vi "获取量程参数存入关键参数.vi"(7 "关键参数变更":bool, 8 "error in (no error)":errorcluster caption="错误输入（无错误）", 9 "量程":u16, 10 "flowid":u16, 11 "id":u16) -> (0 "error out":errorcluster caption="错误输出")   [LabVIEW 2016, in "斯坦道总磷总氮.lvlib"]
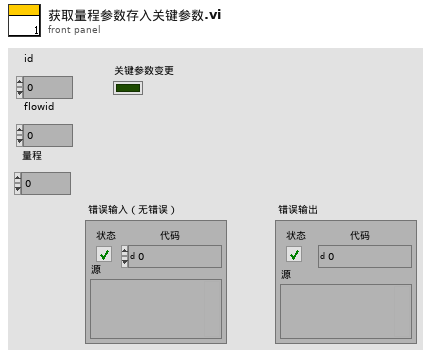
[diagram p1: front panel]
types:
  T1 = cluster{"运行模式":enum16{"维护模式", "常规模式", "应急模式", "质控模式", "性能测试"}, "质控频次":enum16{"关闭", "每天", "星期一", "星期二", "星期三", "星期四", "星期五", "星期六", "星期日"}, "空白核查时间":u16, "跨度核查时间":u16, "测量间隔":u16}
  T2 = cluster{"总磷":dbl, "总氮":dbl, "氨氮":dbl, "磷酸盐":dbl, "硝氮":dbl, "亚硝氮":dbl, "硅酸盐":dbl, "硫化物":dbl, "COD":dbl, "氟化物":dbl, "CODMn":dbl}
  T3 = cluster{"标液浓度1":dbl, "测量吸光度1":dbl, "样品1启用":bool, "标液浓度2":dbl, "测量吸光度2":dbl, "样品2启用":bool, "标液浓度3":dbl, "测量吸光度3":dbl, "样品3启用":bool, "标液浓度4":dbl, "测量吸光度4":dbl, "样品4启用":bool, "标液浓度5":dbl, "测量吸光度5":dbl, "样品5启用":bool, "模型":enum32{"线性", "多项式"}, "精度":dbl, "XY图":cluster{"X Values":dbl[], "Y Values":dbl[]}[], "拟合公式":string, "r^2":dbl, "标样一校准时间":timestamp, "标样二校准时间":timestamp, "标样三校准时间":timestamp, "标样四校准时间":timestamp, "标样五校准时间":timestamp, "二次方程":cluster{"c":dbl, "x":dbl, "x^2":dbl}, "标定时间":timestamp}
  T4 = cluster{"测量精度":u16, "检出限":dbl, "上限":dbl, "下限":dbl, "阈值（低->高）":dbl, "阈值（高->低）":dbl, "稀释度":dbl}
  T5 = typedef "SingleStepTestV3.lvlib/SingleStepTestV3.lvclass/仪器版本.ctl" = enum16{"V3.1版", "V4版", "V3版", "V4.2版"}
  T6 = typedef "斯坦道总磷总氮.lvlib/V3.1版外设参数.ctl" = cluster{"泵类型":u8, "进样速度":u32, "出样速度":u32, "泵阀量":u8, "阀方向":u8, "光谱仪类型":u8, "光谱采样次数":u8, "氙灯次数":u8, "B":u16, "C":u16, "D":u16, "E":u16, "B_COD":u16, "C_COD":u16, "D_COD":u16, "E_COD":u16, "G":u16, "M":u16, "N":u16, "氨氮注射泵控温下限":sgl, "氨氮注射泵控温上限":sgl, "总氮注射泵控温下限":sgl, "总氮注射泵控温上限":sgl, "消解温度下限":sgl, "消解温度上限":sgl, "加热10s限值":sgl, "KP":sgl, "KI":sgl, "KD":sgl, "高温高压阀开阀温度":sgl, "总氮x公式0":u8, "总氮x公式1":sgl, "总氮x公式2":sgl, "总磷浊度稀释系数":sgl, "总磷浊度补偿权重1":sgl, "总磷浊度补偿权重2":sgl, "盐度系数":sgl, "氨氮补偿系数1":sgl, "氨氮补偿系数2":sgl}
  T7 = typedef "斯坦道总磷总氮.lvlib/V4版外设参数.ctl" = cluster{"泵类型":u8, "注射泵正常速度":u32, "注射泵慢速":u32, "阀型号":u8, "res":u8, "光谱仪类型":u8, "光谱采样次数":u8, "氙灯次数":u8, "B":u16, "C":u16, "D":u16, "E":u16, "B_COD":u16, "C_COD":u16, "D_COD":u16, "E_COD":u16, "G":u16, "M":u16, "N":u16, "降温下限":sgl, "降温上限":sgl, "恒温温度下限":sgl, "恒温温度上限":sgl, "消解温度下限":sgl, "消解温度上限":sgl, "加热10s限值":sgl, "KP":sgl, "KI":sgl, "KD":sgl, "高温高压阀开阀温度":sgl, "总氮x公式0":u8, "总氮x公式1":sgl, "总氮x公式2":sgl, "总磷浊度稀释系数":sgl, "总磷浊度补偿权重1":sgl, "总磷浊度补偿权重2":sgl, "盐度系数":sgl, "氨氮补偿系数1":sgl, "氨氮补偿系数2":sgl, "缺试剂传感器阈值":u16}
  T8 = typedef "斯坦道总磷总氮.lvlib/V4.2版外设参数.ctl" = cluster{"工作模式":u16, "泵类型":u16, "阀型号":u16, "注射泵进样速度":u16, "注射泵出样速度":u16, "注射泵滴定速度":u16, "res":u16, "注射泵慢速":u16, "光谱仪类型":u16, "光谱采样次数":u16, "氙灯次数":u16, "B":u16, "C":u16, "D":u16, "E":u16, "B_COD":u16, "C_COD":u16, "D_COD":u16, "E_COD":u16, "G":u16, "M":u16, "N":u16, "温度校准参数":sgl, "降温温度":sgl, "恒温温度":sgl, "消解温度":sgl, "高温高压阀开阀温度":sgl, "加热超时时间":sgl, "KP":sgl, "KI":sgl, "KD":sgl, "消解PID积分上限":sgl, "恒温PID积分上限":sgl, "PID积分下限":sgl, "缺试剂传感器阈值":u16, "滴定延时":u16, "滴定斜率阈值":sgl, "总氮x公式0":u16, "总氮x公式1":sgl, "总氮x公式2":sgl, "总磷浊度稀释系数":sgl, "总磷浊度补偿权重1":sgl, "总磷浊度补偿权重2":sgl, "盐度系数":sgl, "氨氮补偿系数1":sgl, "氨氮补偿系数2":sgl}
  T9 = typedef "斯坦道总磷总氮.lvlib/V3版外设参数.ctl" = cluster{"泵类型":u8, "进样速度":u32, "出样速度":u32, "泵阀量":u8, "光谱仪类型":u8, "光谱采样次数":u8, "氙灯次数":u8, "B":u16, "C":u16, "D":u16, "E":u16, "B_COD":u16, "C_COD":u16, "D_COD":u16, "E_COD":u16, "G":u16, "M":u16, "N":u16, "氨氮注射泵控温下限":sgl, "氨氮注射泵控温上限":sgl, "总氮注射泵控温下限":sgl, "总氮注射泵控温上限":sgl, "消解温度下限":sgl, "消解温度上限":sgl, "加热10s限值":sgl, "高温高压阀开阀温度":sgl, "总氮x公式0":u8, "总氮x公式1":sgl, "总氮x公式2":sgl, "总磷浊度稀释系数":sgl, "总磷浊度补偿权重1":sgl, "总磷浊度补偿权重2":sgl, "盐度系数":sgl, "氨氮补偿系数1":sgl, "氨氮补偿系数2":sgl}
  T10 = cluster{"标液浓度1":dbl, "测量吸光度1":dbl, "样品1启用":bool, "标液浓度2":dbl, "测量吸光度2":dbl, "样品2启用":bool, "标液浓度3":dbl, "测量吸光度3":dbl, "样品3启用":bool, "标液浓度4":dbl, "测量吸光度4":dbl, "样品4启用":bool, "标液浓度5":dbl, "测量吸光度5":dbl, "样品5启用":bool, "模型":enum32{"线性", "多项式"}, "精度":dbl, "XY图":cluster{"X Values":dbl[], "Y Values":dbl[]}[], "拟合公式":string, "r^2":dbl, "标样一校准时间":timestamp, "标样二校准时间":timestamp, "标样三校准时间":timestamp, "标样四校准时间":timestamp, "标样五校准时间":timestamp, "二次方程":cluster{"c":dbl, "x":dbl, "x^2":dbl}, "标定时间":timestamp}[]
  T11 = typedef "斯坦道总磷总氮.lvlib/关键参数.ctl" = cluster{"测量量程":sgl, "测量检出限":sgl, "测量精度":sgl, "测量间隔":sgl, "消解温度":sgl, "消解时长":sgl, "三项式系数":sgl, "二次多项式系数":sgl, "曲线斜率":sgl, "曲线截距":sgl, "线性相关系数":sgl, "空白校准时间":timestamp, "标样校准时间":timestamp, "测量信号值":sgl, "稀释倍数":sgl, "空白标定系数":sgl, "量程系数":sgl}
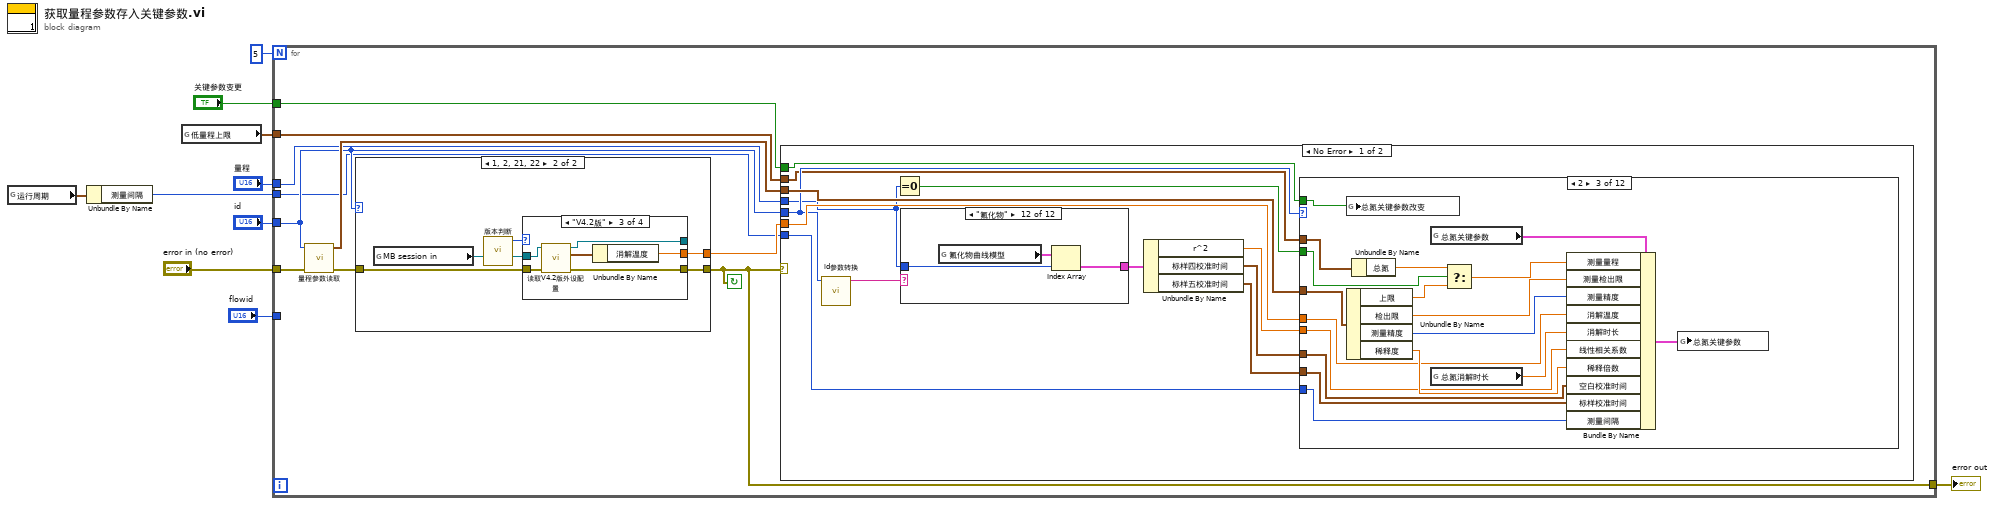
[diagram p0: block diagram]
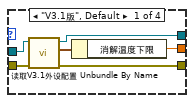
[diagram p3: hidden frame]
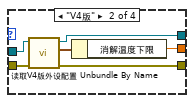
[diagram p4: hidden frame]
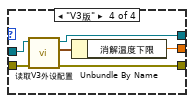
[diagram p5: hidden frame]
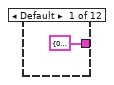
[diagram p6: hidden frame]
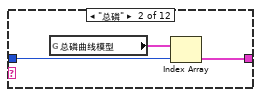
[diagram p7: hidden frame]
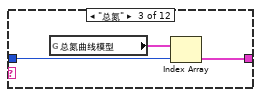
[diagram p8: hidden frame]
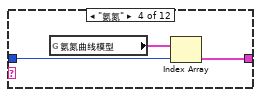
[diagram p9: hidden frame]
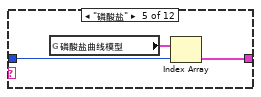
[diagram p10: hidden frame]
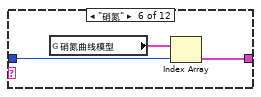
[diagram p11: hidden frame]
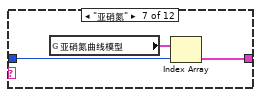
[diagram p12: hidden frame]
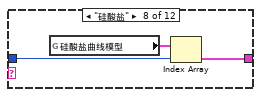
[diagram p13: hidden frame]
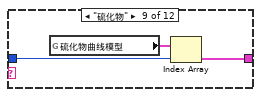
[diagram p14: hidden frame]
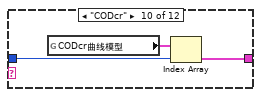
[diagram p15: hidden frame]
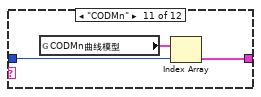
[diagram p16: hidden frame]
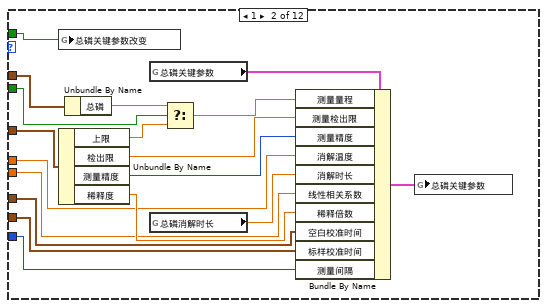
[diagram p18: hidden frame]
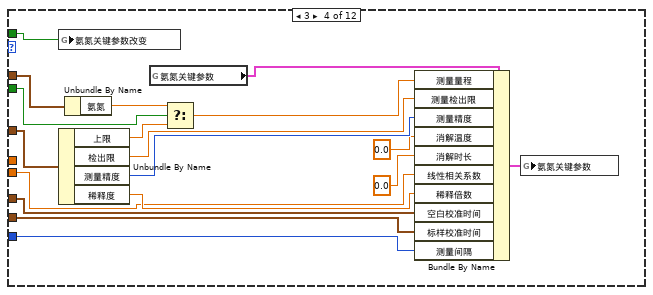
[diagram p19: hidden frame]
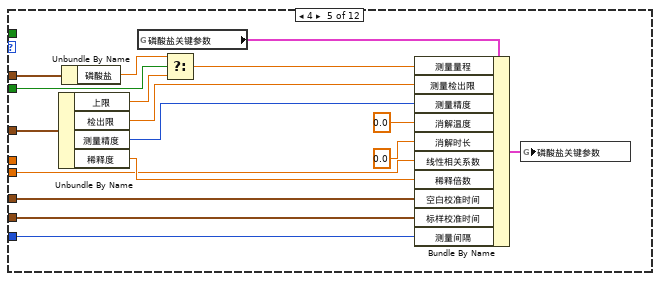
[diagram p20: hidden frame]
diagram:
  n1 = global read "总磷总氮断电保存全局变量.vi" "运行周期"() -> (w4:T1)
  n2 = Unbundle By Name(w4) -> ("测量间隔"=w3:u16)
  n3 = global read "总磷总氮断电保存全局变量.vi" "低量程上限"() -> (w2:T2)
  n4 = for {
    N: 5 -> [_]
    tunnel: "量程" -> [w18]
    tunnel: "flowid" -> [_]
    tunnel: "id" -> [w14]
    tunnel: "error in (no error)" -> [w15]
    tunnel: [w16] -> w5
    tunnel: w3 -> [w13]
    tunnel: w2 -> [w12]
    tunnel: "关键参数变更" -> [w11]
    stop <- w16 continue-if-true
    n5 = call "量程参数读取.vi"("error in (no error)"=w15, "测量参数"=w14) -> ("error out"=w17:errorcluster, "量程参数读取"=w20:T4)  [unwired: 8 in]
    n6 = case shown="1, 2, 21, 22" w14 {
      tunnel: [_ w24] -> w19
      tunnel: w17 -> [w21 w25]
      tunnel: [w21 w23] -> w16
      frame 0, Default {
      }
      frame 1, 2, 21, 22 {
        n7 = global read "VAR总磷总氮全局变量.vi" "MB session in"() -> (w26:refnum<class "MB_Master.lvclass">)
        n8 = call "版本判断.vi"() -> ("仪器版本"=w22:T5)  [unwired: 11 in]
        n9 = case shown="\"V4.2版\"" w22 {
          tunnel: [w32 w38 w44 w50] -> w23
          tunnel: [w30 w36 w42 w48] -> w24
          tunnel: [w29 w35 w41 w47] -> _
          tunnel: w26 -> [w28 w34 w40 w46]
          tunnel: w25 -> [w27 w33 w39 w45]
          frame "V3.1版", Default {
            n10 = call "读取V3.1外设配置.vi"("error in (no error)"=w27, "MB session in"=w28) -> ("error out"=w32:errorcluster, "外设配置"=w31:T6, "MB session out"=w29:refnum<class "MB_Master.lvclass">)  [unwired: 7 in]
            n11 = Unbundle By Name(w31) -> ("消解温度下限"=w30:sgl)
          }
          frame "V4版" {
            n12 = call "读取V4版外设配置.vi"("error in (no error)"=w33, "MB session in"=w34) -> ("error out"=w38:errorcluster, "外设配置"=w37:T7, "MB session out"=w35:refnum<class "MB_Master.lvclass">)  [unwired: 7 in]
            n13 = Unbundle By Name(w37) -> ("消解温度下限"=w36:sgl)
          }
          frame "V4.2版" {
            n14 = call "读取V4.2版外设配置.vi"("error in (no error)"=w39, "MB session in"=w40) -> ("error out"=w44:errorcluster, "外设配置"=w43:T8, "MB session out"=w41:refnum<class "MB_Master.lvclass">)  [unwired: 7 in]
            n15 = Unbundle By Name(w43) -> ("消解温度"=w42:sgl)
          }
          frame "V3版" {
            n16 = call "读取V3外设配置.vi"("error in (no error)"=w45, "MB session in"=w46) -> ("error out"=w50:errorcluster, "外设配置"=w49:T9, "MB session out"=w47:refnum<class "MB_Master.lvclass">)  [unwired: 7 in]
            n17 = Unbundle By Name(w49) -> ("消解温度下限"=w48:sgl)
          }
        }
      }
    }
    n18 = case shown="No Error" w16 {
      tunnel: w20 -> [w63 _]
      tunnel: w19 -> [w62 _]
      tunnel: w14 -> [w56 _]
      tunnel: w18 -> [w53 _]
      tunnel: w13 -> [w55 _]
      tunnel: w12 -> [w54 _]
      tunnel: w11 -> [w51 _]
      frame No Error {
        n19 = call "id参数转换.vi"("id"=w56) -> ("table输出"=w61:string)  [unwired: 9 in, 1 out]
        n20 = Equal To 0?(x=w53) -> (x = 0?=w52:bool)
        n21 = case shown="\"氟化物\"" w61 {
          tunnel: w53 -> [_ w65 w68 w71 w74 w77 w80 w83 w86 w89 w92 w95]
          tunnel: [T3 {"标液浓度1"=0.0, "测量吸光度1"=0.0, "样品1启用"=FALSE, "标液浓度2"=0.0, "测量吸光度2"=0.0, "样品2启用"=FALSE, "标液浓度3"=0.0, "测量吸光度3"=0.0, "样品3启用"=FALSE, "标液浓度4"=0.0, "测量吸光度4"=0.0, "样品4启用"=FALSE, "标液浓度5"=0.0, "测量吸光度5"=0.0, "样品5启用"=FALSE, "模型"=enum."线性", "精度"=0.0, "XY图"=[], "拟合公式"="", "r^2"=0.0, "标样一校准时间"=timestamp(0 s since 1904-01-01), "标样二校准时间"=timestamp(0 s since 1904-01-01), "标样三校准时间"=timestamp(0 s since 1904-01-01), "标样四校准时间"=timestamp(0 s since 1904-01-01), "标样五校准时间"=timestamp(0 s since 1904-01-01), "二次方程"={"c"=0.0, "x"=0.0, "x^2"=0.0}, "标定时间"=timestamp(0 s since 1904-01-01)} ("总磷曲线模型") w66 w69 w72 w75 w78 w81 w84 w87 w90 w93 w96] -> w60
          frame Default {
          }
          frame "总磷" {
            n22 = global read "校准数据全局变量.vi" "总磷曲线模型"() -> (w67:T10)
            n23 = Index Array(array=w67, index=w65) -> (element=w66:T3)
          }
          frame "总氮" {
            n24 = global read "校准数据全局变量.vi" "总氮曲线模型"() -> (w70:T10)
            n25 = Index Array(array=w70, index=w68) -> (element=w69:T3)
          }
          frame "氨氮" {
            n26 = global read "校准数据全局变量.vi" "氨氮曲线模型"() -> (w73:T10)
            n27 = Index Array(array=w73, index=w71) -> (element=w72:T3)
          }
          frame "磷酸盐" {
            n28 = global read "校准数据全局变量.vi" "磷酸盐曲线模型"() -> (w76:T10)
            n29 = Index Array(array=w76, index=w74) -> (element=w75:T3)
          }
          frame "硝氮" {
            n30 = global read "校准数据全局变量.vi" "硝氮曲线模型"() -> (w79:T10)
            n31 = Index Array(array=w79, index=w77) -> (element=w78:T3)
          }
          frame "亚硝氮" {
            n32 = global read "校准数据全局变量.vi" "亚硝氮曲线模型"() -> (w82:T10)
            n33 = Index Array(array=w82, index=w80) -> (element=w81:T3)
          }
          frame "硅酸盐" {
            n34 = global read "校准数据全局变量.vi" "硅酸盐曲线模型"() -> (w85:T10)
            n35 = Index Array(array=w85, index=w83) -> (element=w84:T3)
          }
          frame "硫化物" {
            n36 = global read "校准数据全局变量.vi" "硫化物曲线模型"() -> (w88:T10)
            n37 = Index Array(array=w88, index=w86) -> (element=w87:T3)
          }
          frame "CODcr" {
            n38 = global read "校准数据全局变量.vi" "CODcr曲线模型"() -> (w91:T10)
            n39 = Index Array(array=w91, index=w89) -> (element=w90:T3)
          }
          frame "CODMn" {
            n40 = global read "校准数据全局变量.vi" "CODMn曲线模型"() -> (w94:T10)
            n41 = Index Array(array=w94, index=w92) -> (element=w93:T3)
          }
          frame "氟化物" {
            n42 = global read "校准数据全局变量.vi" "氟化物曲线模型"() -> (w97:T10)
            n43 = Index Array(array=w97, index=w95) -> (element=w96:T3)
          }
        }
        n44 = Unbundle By Name(w60) -> ("r^2"=w59:dbl, "标样四校准时间"=w58:timestamp, "标样五校准时间"=w57:timestamp)
        n45 = case shown="2" w56 {
          tunnel: w63 -> [_ w113 w131 w149 w166 w183 w200 w217 w234 w252 w270 w287]
          tunnel: w62 -> [_ w98 w116 _ _ _ _ _ _ w237 w255 w273]
          tunnel: w59 -> [_ w106 w126 w143 w158 w177 w194 w211 w226 w247 w265 w282]
          tunnel: w58 -> [_ w107 w125 w142 w160 w176 w193 w210 w228 w246 w264 w281]
          tunnel: w57 -> [_ w108 w124 w141 w159 w175 w192 w209 w227 w245 w263 w280]
          tunnel: w55 -> [_ w105 w123 w140 w157 w174 w191 w208 w225 w244 w262 w279]
          tunnel: w54 -> [_ w104 w121 w138 w155 w172 w189 w205 w223 w242 w260 w277]
          tunnel: w52 -> [_ w102 w120 w137 w154 w171 w188 w206 w222 w241 w259 w276]
          tunnel: w51 -> [_ w99 w117 w134 _ _ _ _ _ w238 w256 _]
          frame 0, Default {
          }
          frame 1 {
            n46 = global write "VAR总磷总氮全局变量.vi" "总磷关键参数改变"(w99) -> ()
            n47 = Unbundle By Name(w113) -> ("上限"=w101:dbl, "检出限"=w112:dbl, "测量精度"=w111:u16, "稀释度"=w109:dbl)
            n48 = Unbundle By Name(w104) -> ("总磷"=w103:dbl)
            n49 = global read "VAR总磷总氮全局变量.vi" "总磷关键参数"() -> (w114:T11)
            n50 = global read "总磷总氮断电保存全局变量.vi" "总磷消解时长"() -> (w110:dbl)
            n51 = Select(t=w103, s=w102, f=w101) -> (s? t:f=w100:dbl)
            n52 = Bundle By Name(cluster=w114, "测量量程"=w100, "测量检出限"=w112, "测量精度"=w111, "消解温度"=w98, "消解时长"=w110, "线性相关系数"=w106, "稀释倍数"=w109, "空白校准时间"=w107, "标样校准时间"=w108, "测量间隔"=w105) -> (w115:T11)
            n53 = global write "VAR总磷总氮全局变量.vi" "总磷关键参数"(w115) -> ()
          }
          frame 2 {
            n54 = global write "VAR总磷总氮全局变量.vi" "总氮关键参数改变"(w117) -> ()
            n55 = Unbundle By Name(w131) -> ("上限"=w119:dbl, "检出限"=w130:dbl, "测量精度"=w129:u16, "稀释度"=w127:dbl)
            n56 = Unbundle By Name(w121) -> ("总氮"=w122:dbl)
            n57 = global read "VAR总磷总氮全局变量.vi" "总氮关键参数"() -> (w132:T11)
            n58 = global read "总磷总氮断电保存全局变量.vi" "总氮消解时长"() -> (w128:dbl)
            n59 = Select(t=w122, s=w120, f=w119) -> (s? t:f=w118:dbl)
            n60 = Bundle By Name(cluster=w132, "测量量程"=w118, "测量检出限"=w130, "测量精度"=w129, "消解温度"=w116, "消解时长"=w128, "线性相关系数"=w126, "稀释倍数"=w127, "空白校准时间"=w125, "标样校准时间"=w124, "测量间隔"=w123) -> (w133:T11)
            n61 = global write "VAR总磷总氮全局变量.vi" "总氮关键参数"(w133) -> ()
          }
          frame 3 {
            n62 = global write "VAR总磷总氮全局变量.vi" "氨氮关键参数改变"(w134) -> ()
            n63 = Unbundle By Name(w149) -> ("上限"=w136:dbl, "检出限"=w148:dbl, "测量精度"=w147:u16, "稀释度"=w146:dbl)
            n64 = Unbundle By Name(w138) -> ("氨氮"=w139:dbl)
            n65 = global read "VAR总磷总氮全局变量.vi" "氨氮关键参数"() -> (w150:T11)
            n66 = Select(t=w139, s=w137, f=w136) -> (s? t:f=w135:dbl)
            n67 = Bundle By Name(cluster=w150, "测量量程"=w135, "测量检出限"=w148, "测量精度"=w147, "消解温度"=sgl 0.0, "消解时长"=sgl 0.0, "线性相关系数"=w143, "稀释倍数"=w146, "空白校准时间"=w142, "标样校准时间"=w141, "测量间隔"=w140) -> (w151:T11)
            n68 = global write "VAR总磷总氮全局变量.vi" "氨氮关键参数"(w151) -> ()
          }
          frame 4 {
            n69 = Unbundle By Name(w166) -> ("上限"=w153:dbl, "检出限"=w165:dbl, "测量精度"=w164:u16, "稀释度"=w163:dbl)
            n70 = Unbundle By Name(w155) -> ("磷酸盐"=w156:dbl)
            n71 = global read "VAR总磷总氮全局变量.vi" "磷酸盐关键参数"() -> (w167:T11)
            n72 = Select(t=w156, s=w154, f=w153) -> (s? t:f=w152:dbl)
            n73 = Bundle By Name(cluster=w167, "测量量程"=w152, "测量检出限"=w165, "测量精度"=w164, "消解温度"=sgl 0.0, "消解时长"=sgl 0.0, "线性相关系数"=w158, "稀释倍数"=w163, "空白校准时间"=w160, "标样校准时间"=w159, "测量间隔"=w157) -> (w168:T11)
            n74 = global write "VAR总磷总氮全局变量.vi" "磷酸盐关键参数"(w168) -> ()
          }
          frame 5 {
            n75 = Unbundle By Name(w183) -> ("上限"=w170:dbl, "检出限"=w182:dbl, "测量精度"=w181:u16, "稀释度"=w180:dbl)
            n76 = Unbundle By Name(w172) -> ("硝氮"=w173:dbl)
            n77 = global read "VAR总磷总氮全局变量.vi" "硝氮关键参数"() -> (w184:T11)
            n78 = Select(t=w173, s=w171, f=w170) -> (s? t:f=w169:dbl)
            n79 = Bundle By Name(cluster=w184, "测量量程"=w169, "测量检出限"=w182, "测量精度"=w181, "消解温度"=sgl 0.0, "消解时长"=sgl 0.0, "线性相关系数"=w177, "稀释倍数"=w180, "空白校准时间"=w176, "标样校准时间"=w175, "测量间隔"=w174) -> (w185:T11)
            n80 = global write "VAR总磷总氮全局变量.vi" "硝氮关键参数"(w185) -> ()
          }
          frame 6 {
            n81 = Unbundle By Name(w200) -> ("上限"=w187:dbl, "检出限"=w199:dbl, "测量精度"=w198:u16, "稀释度"=w197:dbl)
            n82 = Unbundle By Name(w189) -> ("亚硝氮"=w190:dbl)
            n83 = global read "VAR总磷总氮全局变量.vi" "亚硝氮关键参数"() -> (w201:T11)
            n84 = Select(t=w190, s=w188, f=w187) -> (s? t:f=w186:dbl)
            n85 = Bundle By Name(cluster=w201, "测量量程"=w186, "测量检出限"=w199, "测量精度"=w198, "消解温度"=sgl 0.0, "消解时长"=sgl 0.0, "线性相关系数"=w194, "稀释倍数"=w197, "空白校准时间"=w193, "标样校准时间"=w192, "测量间隔"=w191) -> (w202:T11)
            n86 = global write "VAR总磷总氮全局变量.vi" "亚硝氮关键参数"(w202) -> ()
          }
          frame 7 {
            n87 = Unbundle By Name(w217) -> ("上限"=w204:dbl, "检出限"=w216:dbl, "测量精度"=w215:u16, "稀释度"=w214:dbl)
            n88 = Unbundle By Name(w205) -> ("硅酸盐"=w207:dbl)
            n89 = global read "VAR总磷总氮全局变量.vi" "硅酸盐关键参数"() -> (w218:T11)
            n90 = Select(t=w207, s=w206, f=w204) -> (s? t:f=w203:dbl)
            n91 = Bundle By Name(cluster=w218, "测量量程"=w203, "测量检出限"=w216, "测量精度"=w215, "消解温度"=sgl 0.0, "消解时长"=sgl 0.0, "线性相关系数"=w211, "稀释倍数"=w214, "空白校准时间"=w210, "标样校准时间"=w209, "测量间隔"=w208) -> (w219:T11)
            n92 = global write "VAR总磷总氮全局变量.vi" "硅酸盐关键参数"(w219) -> ()
          }
          frame 8 {
            n93 = Unbundle By Name(w234) -> ("上限"=w221:dbl, "检出限"=w233:dbl, "测量精度"=w232:u16, "稀释度"=w231:dbl)
            n94 = Unbundle By Name(w223) -> ("硫化物"=w224:dbl)
            n95 = global read "VAR总磷总氮全局变量.vi" "硫化物关键参数"() -> (w235:T11)
            n96 = Select(t=w224, s=w222, f=w221) -> (s? t:f=w220:dbl)
            n97 = Bundle By Name(cluster=w235, "测量量程"=w220, "测量检出限"=w233, "测量精度"=w232, "消解温度"=sgl 0.0, "消解时长"=sgl 0.0, "线性相关系数"=w226, "稀释倍数"=w231, "空白校准时间"=w228, "标样校准时间"=w227, "测量间隔"=w225) -> (w236:T11)
            n98 = global write "VAR总磷总氮全局变量.vi" "硫化物关键参数"(w236) -> ()
          }
          frame 22 {
            n99 = global write "VAR总磷总氮全局变量.vi" "CODCr关键参数改变"(w238) -> ()
            n100 = Unbundle By Name(w252) -> ("上限"=w240:dbl, "检出限"=w251:dbl, "测量精度"=w250:u16, "稀释度"=w249:dbl)
            n101 = Unbundle By Name(w242) -> ("亚硝氮"=w243:dbl)
            n102 = global read "VAR总磷总氮全局变量.vi" "CODcr关键参数"() -> (w253:T11)
            n103 = global read "总磷总氮断电保存全局变量.vi" "CODcr消解时长"() -> (w248:dbl)
            n104 = Select(t=w243, s=w241, f=w240) -> (s? t:f=w239:dbl)
            n105 = Bundle By Name(cluster=w253, "测量量程"=w239, "测量检出限"=w251, "测量精度"=w250, "消解温度"=w237, "消解时长"=w248, "线性相关系数"=w247, "稀释倍数"=w249, "空白校准时间"=w246, "标样校准时间"=w245, "测量间隔"=w244) -> (w254:T11)
            n106 = global write "VAR总磷总氮全局变量.vi" "CODcr关键参数"(w254) -> ()
          }
          frame 21 {
            n107 = global write "VAR总磷总氮全局变量.vi" "CODmn关键参数改变"(w256) -> ()
            n108 = Unbundle By Name(w270) -> ("上限"=w258:dbl, "检出限"=w269:dbl, "测量精度"=w268:u16, "稀释度"=w267:dbl)
            n109 = Unbundle By Name(w260) -> ("CODMn"=w261:dbl)
            n110 = global read "VAR总磷总氮全局变量.vi" "CODMn关键参数"() -> (w271:T11)
            n111 = global read "总磷总氮断电保存全局变量.vi" "CODmn消解时长"() -> (w266:dbl)
            n112 = Select(t=w261, s=w259, f=w258) -> (s? t:f=w257:dbl)
            n113 = Bundle By Name(cluster=w271, "测量量程"=w257, "测量检出限"=w269, "测量精度"=w268, "消解温度"=w255, "消解时长"=w266, "线性相关系数"=w265, "稀释倍数"=w267, "空白校准时间"=w264, "标样校准时间"=w263, "测量间隔"=w262) -> (w272:T11)
            n114 = global write "VAR总磷总氮全局变量.vi" "CODMn关键参数"(w272) -> ()
          }
          frame 50 {
            n115 = Unbundle By Name(w287) -> ("上限"=w275:dbl, "检出限"=w286:dbl, "测量精度"=w285:u16, "稀释度"=w284:dbl)
            n116 = Unbundle By Name(w277) -> ("氟化物"=w278:dbl)
            n117 = global read "总磷总氮断电保存全局变量.vi" "CODmn消解时长"() -> (w283:dbl)
            n118 = global read "VAR总磷总氮全局变量.vi" "氟化物关键参数"() -> (w288:T11)
            n119 = Select(t=w278, s=w276, f=w275) -> (s? t:f=w274:dbl)
            n120 = Bundle By Name(cluster=w288, "测量量程"=w274, "测量检出限"=w286, "测量精度"=w285, "消解温度"=w273, "消解时长"=w283, "线性相关系数"=w282, "稀释倍数"=w284, "空白校准时间"=w281, "标样校准时间"=w280, "测量间隔"=w279) -> (w289:T11)
            n121 = global write "VAR总磷总氮全局变量.vi" "氟化物关键参数"(w289) -> ()
          }
        }
      }
      frame Error {
      }
    }
  }
  "error out" <- w5
